vi "RollerPneumaticCVCI.vi"(11 "Integer":dbl) -> (3 "CheckValueChangeInt":bool)   [LabVIEW 2013]
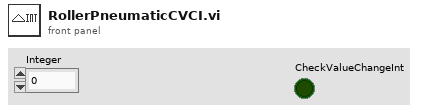
[diagram p1: front panel]
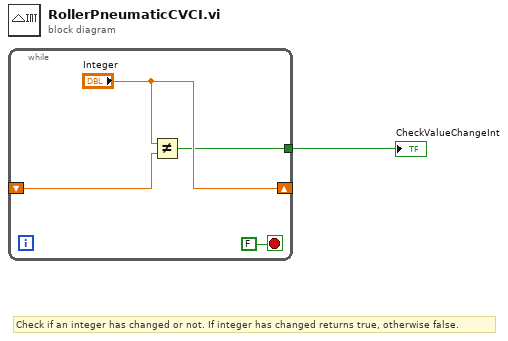
[diagram p0: block diagram]
diagram:
  # "Check if an integer has changed or not. If integer has changed returns true, otherwise false."
  n1 = while {
    shift-right: ["Integer"] -> _
    shift-left: _ -> [w3]
    tunnel: [w2] -> w1
    stop <- FALSE stop-if-true
    n2 = Not Equal?(x="Integer", y=w3) -> (x != y?=w2:bool)
  }
  "CheckValueChangeInt" <- w1
